vi "CleanUp Diagram.vi"(8 "error in (no error)":errorcluster, 10 "Top Level Diagram":refnum<vi>, 11 "DMA Loop in":refnum<class "DMA Loop.lvclass">) -> (0 "error out":errorcluster, 3 "DMA Loop out":refnum<class "DMA Loop.lvclass">)   [LabVIEW 2015, in "DMA Loop.lvclass"]
uses:
  DMA Loop.lvclass
  Structures/Structures.lvclass/Structures.ctl
  DMA Loop.lvclass/DMA Loop.ctl
  Structures/Read Structure.vi
  Read Loop Structure.vi
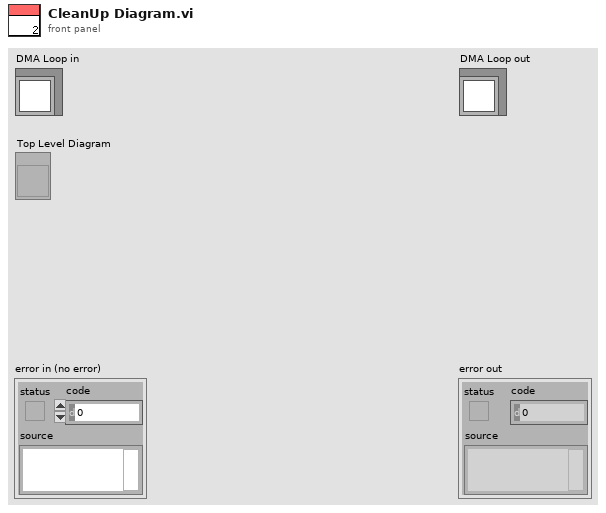
[diagram p1: front panel]
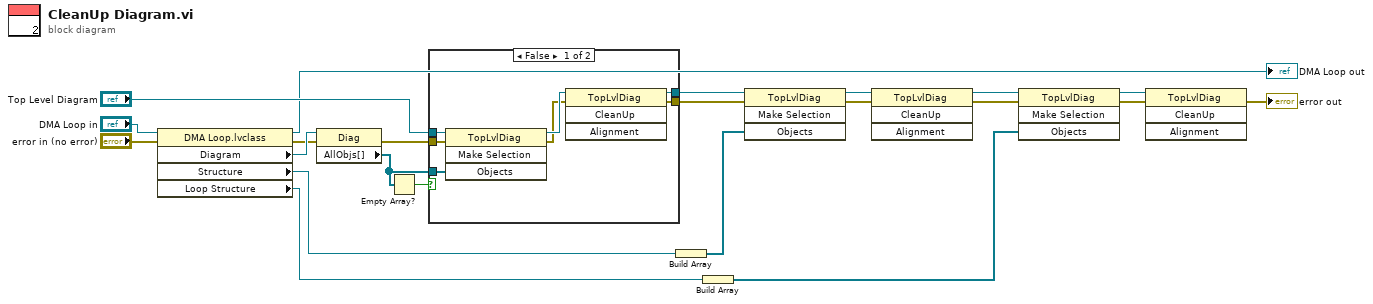
[diagram p0: block diagram]
diagram:
  n1 = property class="DMA Loop.lvclass"(reference="DMA Loop in", error in="error in (no error)") -> (reference out=→"DMA Loop out":refnum<class "DMA Loop.lvclass">, error out=w21:errorcluster, "Diagram"=w22:refnum<vi>, "Structure"=w11:refnum<vi>, "Loop Structure"=w4:refnum<vi>)
  n2 = property class="Diag"(reference=w22, error in=w21) -> (error out=w20:errorcluster, "AllObjs[]"=w15:refnum<vi>[])  [unwired: 1 out]
  n3 = Empty Array?(array=w15) -> (empty?=w14:bool)
  n4 = case shown="False" w14 {
    tunnel: "Top Level Diagram" -> [w29 w30]
    tunnel: w20 -> [w26 w31]
    tunnel: [w25 w31] -> w19
    tunnel: [w24 w30] -> w17
    tunnel: w15 -> [w23 _]
    frame False {
      n5 = invoke class="TopLvlDiag" method="Make Selection"(reference=w29, error in=w26, "Objects"=w23) -> (reference out=w28:refnum<vi>, error out=w27:errorcluster)  [unwired: 1 in, 2 out]
      n6 = invoke class="TopLvlDiag" method="CleanUp"(reference=w28, error in=w27) -> (reference out=w24:refnum<vi>, error out=w25:errorcluster)  [unwired: 2 in, 2 out]
    }
    frame True {
    }
  }
  n7 = Build Array(w11) -> (w9:refnum<vi>[])
  n8 = Build Array(w4) -> (w3:refnum<vi>[])
  n9 = invoke class="TopLvlDiag" method="Make Selection"(reference=w17, error in=w19, "Objects"=w9) -> (reference out=w16:refnum<vi>, error out=w18:errorcluster)  [unwired: 1 in, 2 out]
  n10 = invoke class="TopLvlDiag" method="CleanUp"(reference=w16, error in=w18) -> (reference out=w5:refnum<vi>, error out=w6:errorcluster)  [unwired: 2 in, 2 out]
  n11 = invoke class="TopLvlDiag" method="Make Selection"(reference=w5, error in=w6, "Objects"=w3) -> (reference out=w8:refnum<vi>, error out=w7:errorcluster)  [unwired: 1 in, 2 out]
  n12 = invoke class="TopLvlDiag" method="CleanUp"(reference=w8, error in=w7) -> (error out=→"error out":errorcluster)  [unwired: 2 in, 3 out]
